vi "Redo.vi"(8 "error in (no error)":errorcluster, 11 "Map Model in":refnum<class "Map Model.lvclass">) -> (0 "error out":errorcluster, 3 "Map Model out":refnum<class "Map Model.lvclass">)   [LabVIEW 2020, in "Map Model.lvlib" / "Map Model.lvclass"]
uses:
  Map Model.lvclass
  Map Model.lvclass/Map Model.ctl
  Tools/Undoable Tool/Undoable Tool.lvclass/Undoable Tool.ctl
  Tools/Undoable Tool/Undoable Tool.lvclass
  Stack/Stack.lvclass
panel:
  # "NOTICE -- YOU MUST LEAVE THIS NOTICE IN PLACE.\n\nCopyright (c) 2017, LIANG LIU Shawn.Liu.cn@gmail.com\nAll rights reserved.\n\nRedistribution and use in source and binary forms, with or without modification, are permitted provided that the following conditions are met:\n-Redistributions of source code must retain the above copyright notice, this list of conditions and the following disclaimer.\n-Redistributions in binary form must reproduce the above copyright notice, this list of conditions and the following disclaimer in the documentation and/or other materials provided with the distribution.\n-Neither the name of the eLp nor the names of its contributors may be used to endorse or promote products derived from this software without specific prior written permission.\n\nTHIS SOFTWARE IS PROVIDED BY THE COPYRIGHT HOLDERS AND CONTRIBUTORS \"AS IS\" AND ANY EXPRESS OR IMPLIED WARRANTIES, INCLUDING, BUT NOT LIMITED TO, THE IMPLIED WARRANTIES OF MERCHANTABILITY AND FITNESS FOR A PARTICULAR PURPOSE ARE DISCLAIMED. IN NO EVENT SHALL THE COPYRIGHT HOLDER OR CONTRIBUTORS BE LIABLE FOR ANY DIRECT, INDIRECT, INCIDENTAL, SPECIAL, EXEMPLARY, OR CONSEQUENTIAL DAMAGES (INCLUDING, BUT NOT LIMITED TO, PROCUREMENT OF SUBSTITUTE GOODS OR SERVICES; LOSS OF USE, DATA, OR PROFITS; OR BUSINESS INTERRUPTION) HOWEVER CAUSED AND ON ANY THEORY OF LIABILITY, WHETHER IN CONTRACT, STRICT LIABILITY, OR TORT (INCLUDING NEGLIGENCE OR OTHERWISE) ARISING IN ANY WAY OUT OF THE USE OF THIS SOFTWARE, EVEN IF ADVISED OF THE POSSIBILITY OF SUCH DAMAGE."
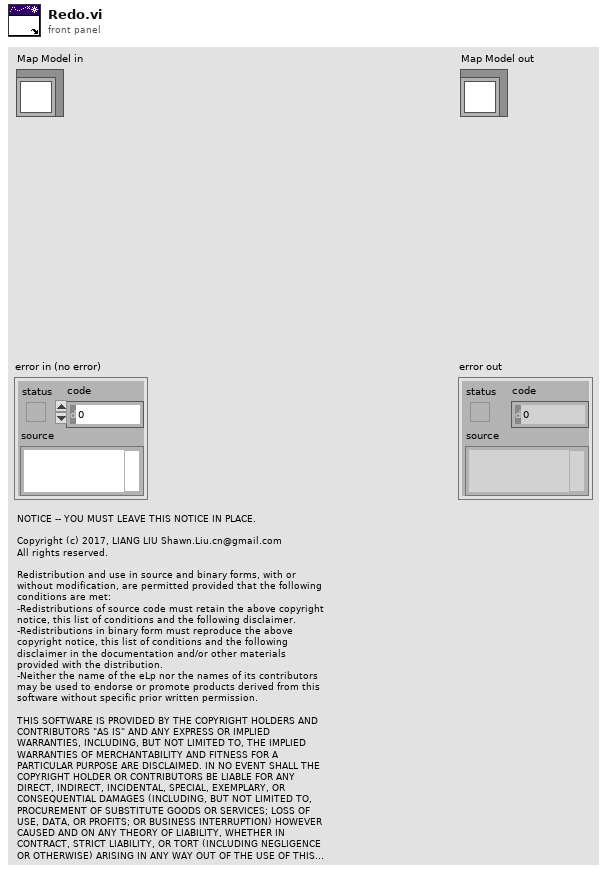
[diagram p1: front panel]
types:
  T1 = enum8{"Enabled", "Disabled", "Disabled and Grayed Out"}
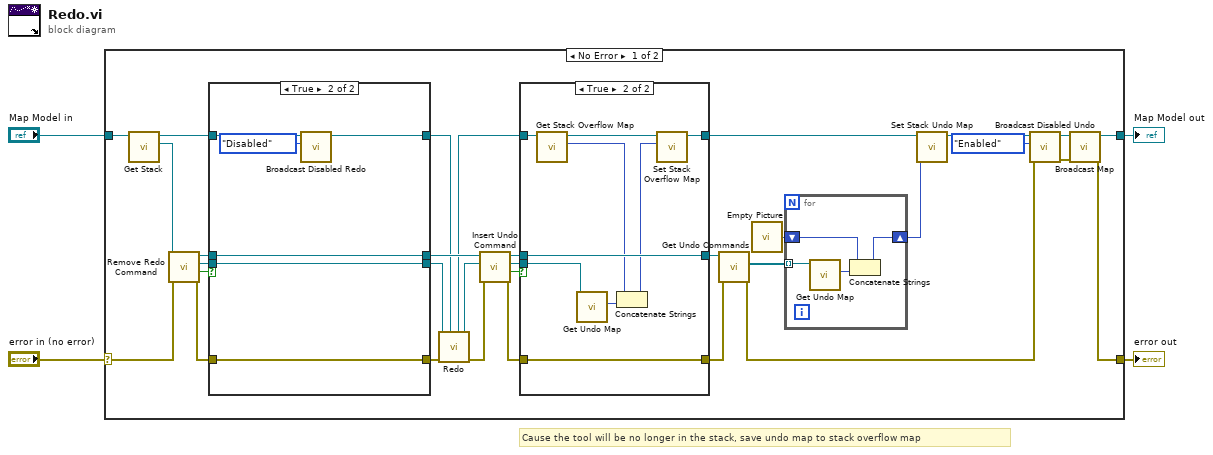
[diagram p0: block diagram]
diagram:
  # "Cause the tool will be no longer in the stack, save undo map to stack overflow map"
  n1 = case shown="No Error" "error in (no error)" {
    selector: "error in (no error)" -> [w35 w64]
    tunnel: "Map Model in" -> [w36 w63]
    tunnel: [w34 w64] -> w2
    tunnel: [w33 w63] -> w1
    frame No Error {
      n2 = call "Get Stack.vi"("Map Model in"=w36) -> ("Stack"=w32:refnum<class "Stack.lvclass">, "Map Model out"=w28:refnum<class "Map Model.lvclass">)  [unwired: 9 in]
      n3 = call "Remove Redo Command.vi"("error in (no error)"=w35, "Stack in"=w32) -> ("error out"=w21:errorcluster, "Empty"=w31:bool, "Redo Command"=w29:refnum<class "Undoable Tool.lvclass">, "Stack out"=w30:refnum<class "Stack.lvclass">)  [unwired: 6 in]
      n4 = case shown="True" w31 {
        tunnel: w30 -> [w56 w61]
        tunnel: w29 -> [w55 w62]
        tunnel: [w55 w62] -> w24
        tunnel: [w56 w61] -> w27
        tunnel: w28 -> [w54 w60]
        tunnel: [w54 w58] -> w22
        tunnel: w21 -> [w53 w59]
        tunnel: [w53 w59] -> w20
        frame False {
        }
        frame True {
          n5 = call "Broadcast Disabled Redo.vi"("Disabled Redo"=T1."Disabled", "Map Model in"=w60) -> ("Map Model out"=w58:refnum<class "Map Model.lvclass">)  [unwired: 8 in, 1 out]
        }
      }
      n6 = call-dynamic "Redo.vi"("Map Model in"=w22, "error in (no error)"=w20, "Undoable Tool in"=w24) -> ("error out"=w18:errorcluster, "Undoable Tool out"=w23:refnum<class "Undoable Tool.lvclass">, "Map Model out"=w17:refnum<class "Map Model.lvclass">)  [unwired: 6 in]
      n7 = call "Insert Undo Command.vi"("error in (no error)"=w18, "Undo Command"=w23, "Stack in"=w27) -> ("error out"=w14:errorcluster, "Overflow"=w11:bool, "Overflow Undo Command"=w15:refnum<class "Undoable Tool.lvclass">, "Stack out"=w16:refnum<class "Stack.lvclass">)  [unwired: 5 in]
      n8 = case shown="True" w11 {
        tunnel: w16 -> [w39 w48]
        tunnel: w15 -> [_ w43]
        tunnel: [w39 w48] -> w12
        tunnel: w17 -> [w38 w47]
        tunnel: [w38 w44] -> w9
        tunnel: w14 -> [w37 w46]
        tunnel: [w37 w46] -> w13
        frame False {
        }
        frame True {
          n9 = call "Get Stack Overflow Map.vi"("Map Model in"=w47) -> ("Stack Overflow Map"=w41:picture, "Map Model out"=w45:refnum<class "Map Model.lvclass">)  [unwired: 9 in]
          n10 = call "Get Undo Map.vi"("Undoable Tool in"=w43) -> ("Undo Map"=w42:picture)  [unwired: 9 in, 1 out]
          n11 = Concatenate Strings(w41, w42) -> (w40:picture)
          n12 = call "Set Stack Overflow Map.vi"("Stack Overflow Map"=w40, "Map Model in"=w45) -> ("Map Model out"=w44:refnum<class "Map Model.lvclass">)  [unwired: 9 in]
        }
      }
      n13 = call "Get Undo Commands.vi"("error in (no error)"=w13, "Stack in"=w12) -> ("error out"=w6:errorcluster, "Undo Commands"=w26:refnum<class "Undoable Tool.lvclass">[])  [unwired: 7 in, 1 out]
      n14 = call "Empty Picture"() -> ("empty picture"=w25:picture)
      n15 = for {
        tunnel: w26 -> [w52] mode=indexing
        shift-right: [w49] -> w19
        shift-left: w25 -> [w50]
        n16 = call "Get Undo Map.vi"("Undoable Tool in"=w52) -> ("Undo Map"=w51:picture)  [unwired: 9 in, 1 out]
        n17 = Concatenate Strings(w50, w51) -> (w49:picture)
      }
      n18 = call "Set Stack Undo Map.vi"("Stack Undo Map"=w19, "Map Model in"=w9) -> ("Map Model out"=w8:refnum<class "Map Model.lvclass">)  [unwired: 9 in]
      n19 = call "Broadcast Disabled Undo.vi"("error in (no error)"=w6, "Disabled Undo"=T1."Enabled", "Map Model in"=w8) -> ("error out"=w5:errorcluster, "Map Model out"=w7:refnum<class "Map Model.lvclass">)  [unwired: 7 in]
      n20 = call "Broadcast Map.vi"("error in (no error)"=w5, "Map Model in"=w7) -> ("error out"=w34:errorcluster, "Map Model out"=w33:refnum<class "Map Model.lvclass">)  [unwired: 8 in]
    }
    frame Error {
    }
  }
  "error out" <- w2
  "Map Model out" <- w1
